vi "hotSpotsFinder.vi"(3 "y":i32, 4 "x":i32, 5 "Basket Number":i32) -> (0 "in Hotspot":bool, 1 "rotation angle":dbl, 2 "distance to basket":dbl)   [LabVIEW 2011]
panel:
  # "2"
  # "1, 4"
  # "3"
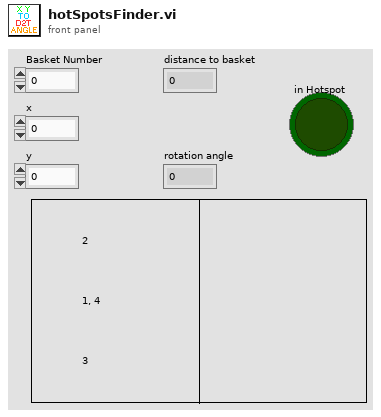
[diagram p1: front panel]
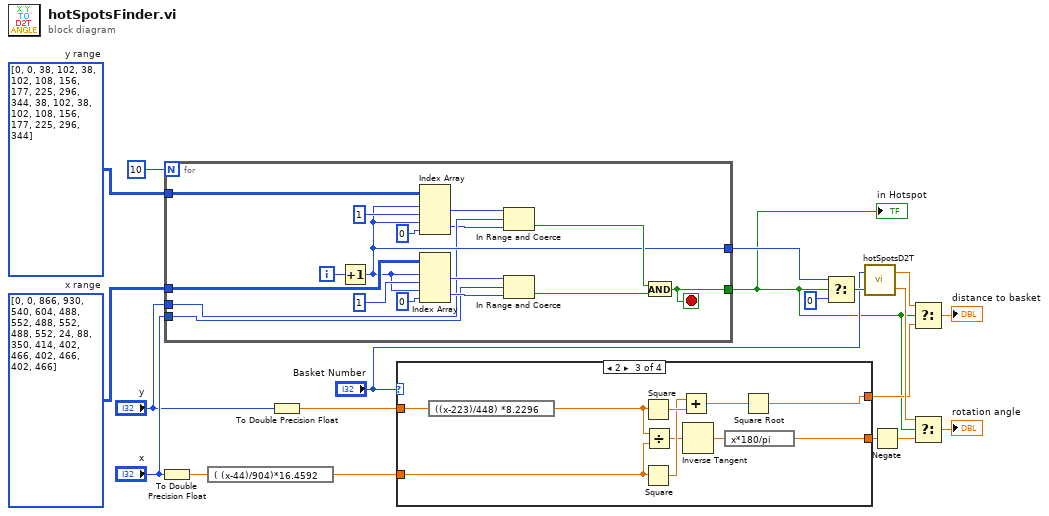
[diagram p0: block diagram]
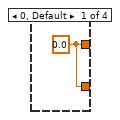
[diagram p2: hidden frame]
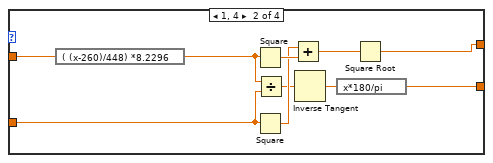
[diagram p3: hidden frame]
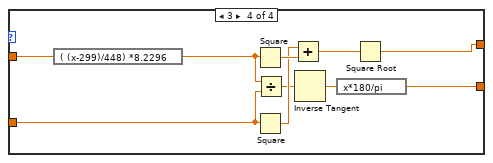
[diagram p4: hidden frame]
diagram:
  w18 = i32[][] [[0, 0], [38, 102], [38, 102], [108, 156], [177, 225], [296, 344], [38, 102], [38, 102], [108, 156], [177, 225], [296, 344]]  # y range
  w19 = i32[][] [[0, 0], [866, 930], [540, 604], [488, 552], [488, 552], [488, 552], [24, 88], [350, 414], [402, 466], [402, 466], [402, 466]]  # x range
  n1 = To Double Precision Float(number="x") -> (double precision float=w9:dbl)
  n2 = for {
    N: 10 -> [_]
    tunnel: w19 -> [w37]
    tunnel: "x" -> [w31]
    tunnel: [w26] -> w17
    tunnel: [w21] -> w2
    tunnel: w18 -> [w25]
    tunnel: "y" -> [w24]
    i -> [w36]
    stop <- w21 stop-if-true
    n3 = Increment(x=w36) -> (x+1=w26:i32)
    n4 = Index Array(array=w25, index (row) #1=w26, index (col) #1=1 ("disabled index (col)"), index (row) #2=w26, index (col) #2=0 ("disabled index (col)")) -> (element #1=w23:i32, element #2=w22:i32)
    n5 = Index Array(array=w37, index (row) #1=w26, index (col) #1=1 ("disabled index (col)"), index (row) #2=w26, index (col) #2=0 ("disabled index (col)")) -> (element #1=w32:i32, element #2=w33:i32)
    n6 = In Range and Coerce(upper limit=w23, x=w24, lower limit=w22) -> (In Range?=w27:bool)  [unwired: 1 out]
    n7 = In Range and Coerce(upper limit=w32, x=w31, lower limit=w33) -> (In Range?=w28:bool)  [unwired: 1 out]
    n8 = And(x=w27, y=w28) -> (x .and. y?=w21:bool)
  }
  "in Hotspot" <- w2
  n9 = expression code="( (x-44)/904)*16.4592"(w9) -> (w5:dbl)
  n10 = To Double Precision Float(number="y") -> (double precision float=w6:dbl)
  n11 = case shown="2" "Basket Number" {
    tunnel: [w38 w44 w49 w59] -> w4
    tunnel: w6 -> [_ w48 w51 w61]
    tunnel: w5 -> [_ w40 w52 w62]
    tunnel: [w38 w42 w50 w60] -> w3
    frame 0, Default {
      w38 = 0.0 ("z")
    }
    frame 1, 4 {
      n12 = expression code="( (x-260)/448) *8.2296"(w48) -> (w41:dbl)
      n13 = Square(x=w41) -> (x^2=w47:dbl)
      n14 = Square(x=w40) -> (x^2=w46:dbl)
      n15 = Divide(x=w41, y=w40) -> (x/y=w39:dbl)
      n16 = Add(x=w46, y=w47) -> (x+y=w45:dbl)
      n17 = Inverse Tangent(1:w39) -> (0:w43:dbl)
      n18 = expression code="x*180/pi"(w43) -> (w42:dbl)
      n19 = Square Root(x=w45) -> (sqrt(x)=w44:dbl)
    }
    frame 2 {
      n20 = expression code="((x-223)/448) *8.2296"(w51) -> (w54:dbl)
      n21 = Square(x=w54) -> (x^2=w58:dbl)
      n22 = Square(x=w52) -> (x^2=w57:dbl)
      n23 = Divide(x=w54, y=w52) -> (x/y=w53:dbl)
      n24 = Add(x=w57, y=w58) -> (x+y=w56:dbl)
      n25 = Inverse Tangent(1:w53) -> (0:w55:dbl)
      n26 = expression code="x*180/pi"(w55) -> (w50:dbl)
      n27 = Square Root(x=w56) -> (sqrt(x)=w49:dbl)
    }
    frame 3 {
      n28 = expression code="( (x-299)/448) *8.2296"(w61) -> (w64:dbl)
      n29 = Square(x=w64) -> (x^2=w68:dbl)
      n30 = Square(x=w62) -> (x^2=w67:dbl)
      n31 = Divide(x=w64, y=w62) -> (x/y=w63:dbl)
      n32 = Add(x=w67, y=w68) -> (x+y=w66:dbl)
      n33 = Inverse Tangent(1:w63) -> (0:w65:dbl)
      n34 = expression code="x*180/pi"(w65) -> (w60:dbl)
      n35 = Square Root(x=w66) -> (sqrt(x)=w59:dbl)
    }
  }
  n36 = Select(t=w17, s=w2, f=0) -> (s? t:f=w15:i32)
  n37 = call "hotSpotsD2T.vi"("Hotspot Number"=w15, "Basket Number"="Basket Number") -> ("rotation angle"=w12:dbl, "distance to basket"=w11:dbl)
  n38 = Negate(x=w3) -> (-x=w1:dbl)
  n39 = Select(t=w11, s=w2, f=w4) -> (s? t:f=→"distance to basket":dbl)
  n40 = Select(t=w12, s=w2, f=w1) -> (s? t:f=→"rotation angle":dbl)
